vi "Is VI Running Top Level.vi"() -> (1 "Top Level?":bool)   [LabVIEW 2023]
doc: "Is current VI running top level. If False, then it is called by another VI."
panel:
  out "call chain size":i32
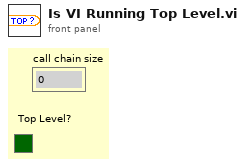
[diagram p1: front panel]
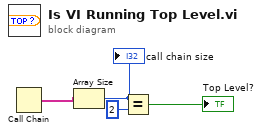
[diagram p0: block diagram]
diagram:
  n1 = Call Chain() -> (call chain=w4:string[])
  n2 = Array Size(array=w4) -> (size(s)=w3:i32)
  "call chain size" <- w3
  n3 = Equal?(x=w3, y=2) -> (x = y?=→"Top Level?":bool)
